vi "power_supply_main.vi"(6 "Enable Output (T: Enable)":bool=TRUE, 8 "error in (no error)":errorcluster, 9 "command":string, 10 "channel":i32, 11 "VISA resource name":refnum<visa-resource-name>) -> (0 "error out":errorcluster, 3 "VISA resource name out":refnum<visa-resource-name>)   [LabVIEW 2020]
uses:
  <instrlib>/GPD-3303/GPD-3303.lvlib
panel:
  # "{\"number of process\": 1, \"experiment_No\": 1, \"process1\": {\"1\": {\"device\": \"power_supply2\", \"operation\": {\"ID\": 3, \"command\": \"2.62\"}}, \"2\": {\"device\": \"wait3\", \"operation\": 1.0}, \"3\": {\"device\": \"power_supply2\", \"operation\": {\"ID\": 3, \"command\": \"0\"}}, \"number of steps\": 3}}"
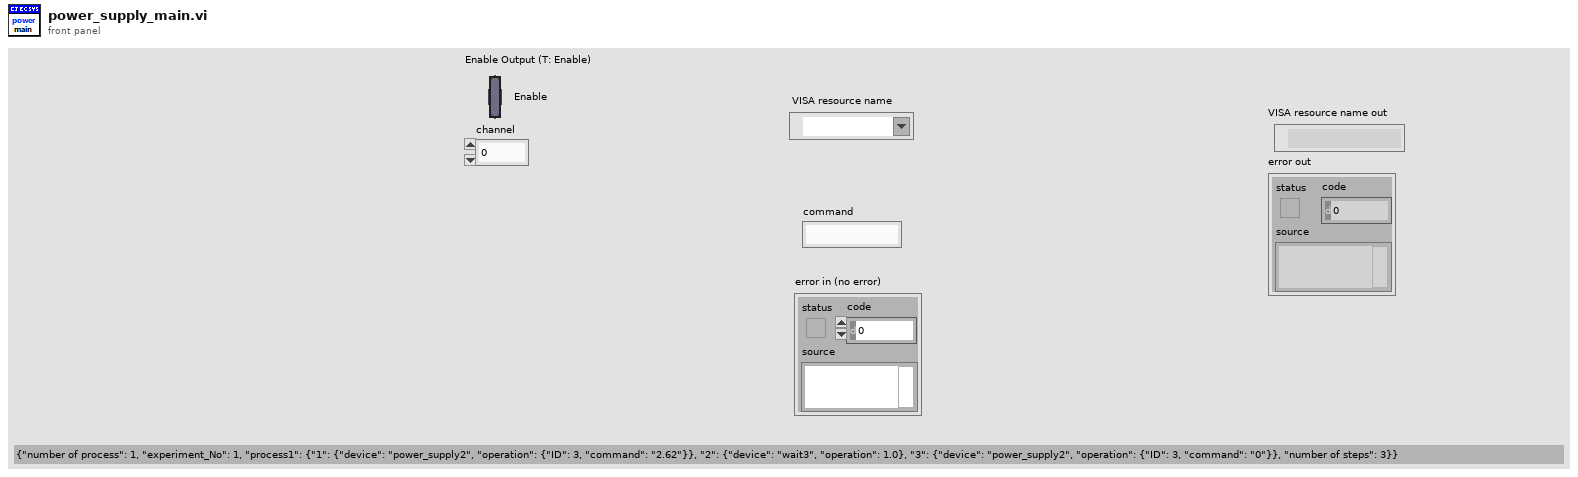
[diagram p1: front panel]
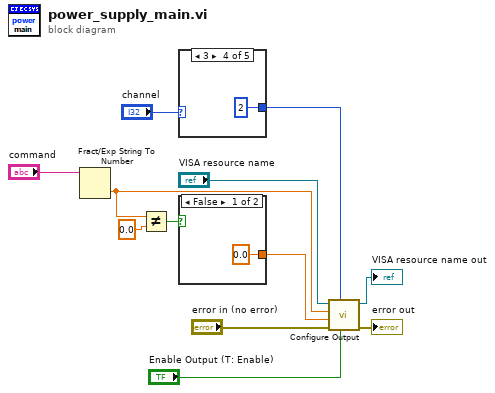
[diagram p0: block diagram]
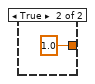
[diagram p2: hidden frame]
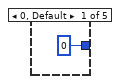
[diagram p3: hidden frame]
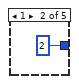
[diagram p4: hidden frame]
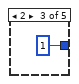
[diagram p5: hidden frame]
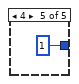
[diagram p6: hidden frame]
diagram:
  n1 = Fract/Exp String To Number(string="command") -> (number=w1:dbl)  [unwired: 3 in, 1 out]
  n2 = Not Equal?(x=w1, y=0.0) -> (x != y?=w4:bool)
  n3 = case shown="3" "channel" {
    tunnel: [0 ("Channel (1: Channel 1)") 2 ("Channel (1: Channel 1)") 1 ("Channel (1: Channel 1)") 2 ("Channel (1: Channel 1)") 1 ("Channel (1: Channel 1)")] -> w12
    frame 0, Default {
    }
    frame 1 {
    }
    frame 2 {
    }
    frame 3 {
    }
    frame 4 {
    }
  }
  n4 = case shown="False" w4 {
    tunnel: [0.0 ("Current Level (0.0 V)") 1.0 ("Current Level (0.0 V)")] -> w3
    frame False {
    }
    frame True {
    }
  }
  n5 = call <instrlib>:"Configure Output.vi"("Enable Output (T: Enable)"="Enable Output (T: Enable)", "Channel (1: Channel 1)"=w12, "error in (no error)"="error in (no error)", "Current Level (0.0 V)"=w3, "Voltage Level (0.0 V)"=w1, "VISA resource name"="VISA resource name") -> ("error out"=→"error out":errorcluster, "VISA resource name out"=→"VISA resource name out":refnum<visa-resource-name>)  [unwired: 4 in]
